vi "UpdateGraphV2.vi"(8 "error in (no error)":errorcluster caption="entrée d'erreur (pas d'erreur)", 10 "GraphIndexArr":i32[](array[numeric]), 11 "Interface en entrée":refnum<class "Interface.lvclass"> caption="DNL_LabVIEW Object in") -> (0 "error out":errorcluster caption="sortie d'erreur", 3 "Interface en sortie":refnum<class "Interface.lvclass"> caption="DNL_LabVIEW Object out")   [LabVIEW 2012, in "Interface.lvclass"]
uses:
  Interface.lvclass
  Interface.lvclass/Interface.ctl
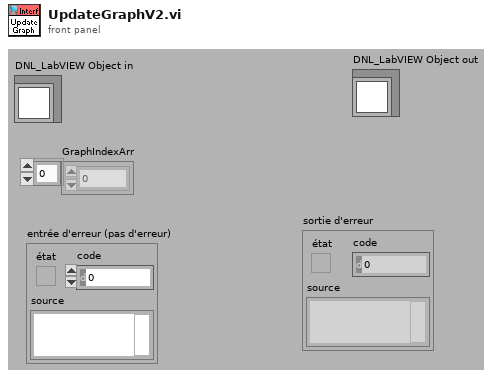
[diagram p1: front panel]
types:
  T1 = typedef "Interface.lvclass/CurveSetup.ctl" = cluster{"CurveName":string, "YParam":string, "XParam":string, "ZParam ":string, "GroupName":string, "LinWdth":u8, "PntCol":u32, "LinCol":u32, "LablFor":u8, "XScale":u32, "YScale":u32, "Interpol":u8, "DisplayName":string, "FillType":i16, "LineStyle":u8, "PntStyle":u8, "BarTyp":u8, "GraphIndex":i32, "Visible":bool, "XScaleName":string, "YScaleName":string, "XYGraph_Ref":refnum<vi>, "Data Only":bool, "DataQ Ref":refnum<queue>, "XParQ Ref":refnum<queue>, "XParamInd":i32, "ScanInd":i32}
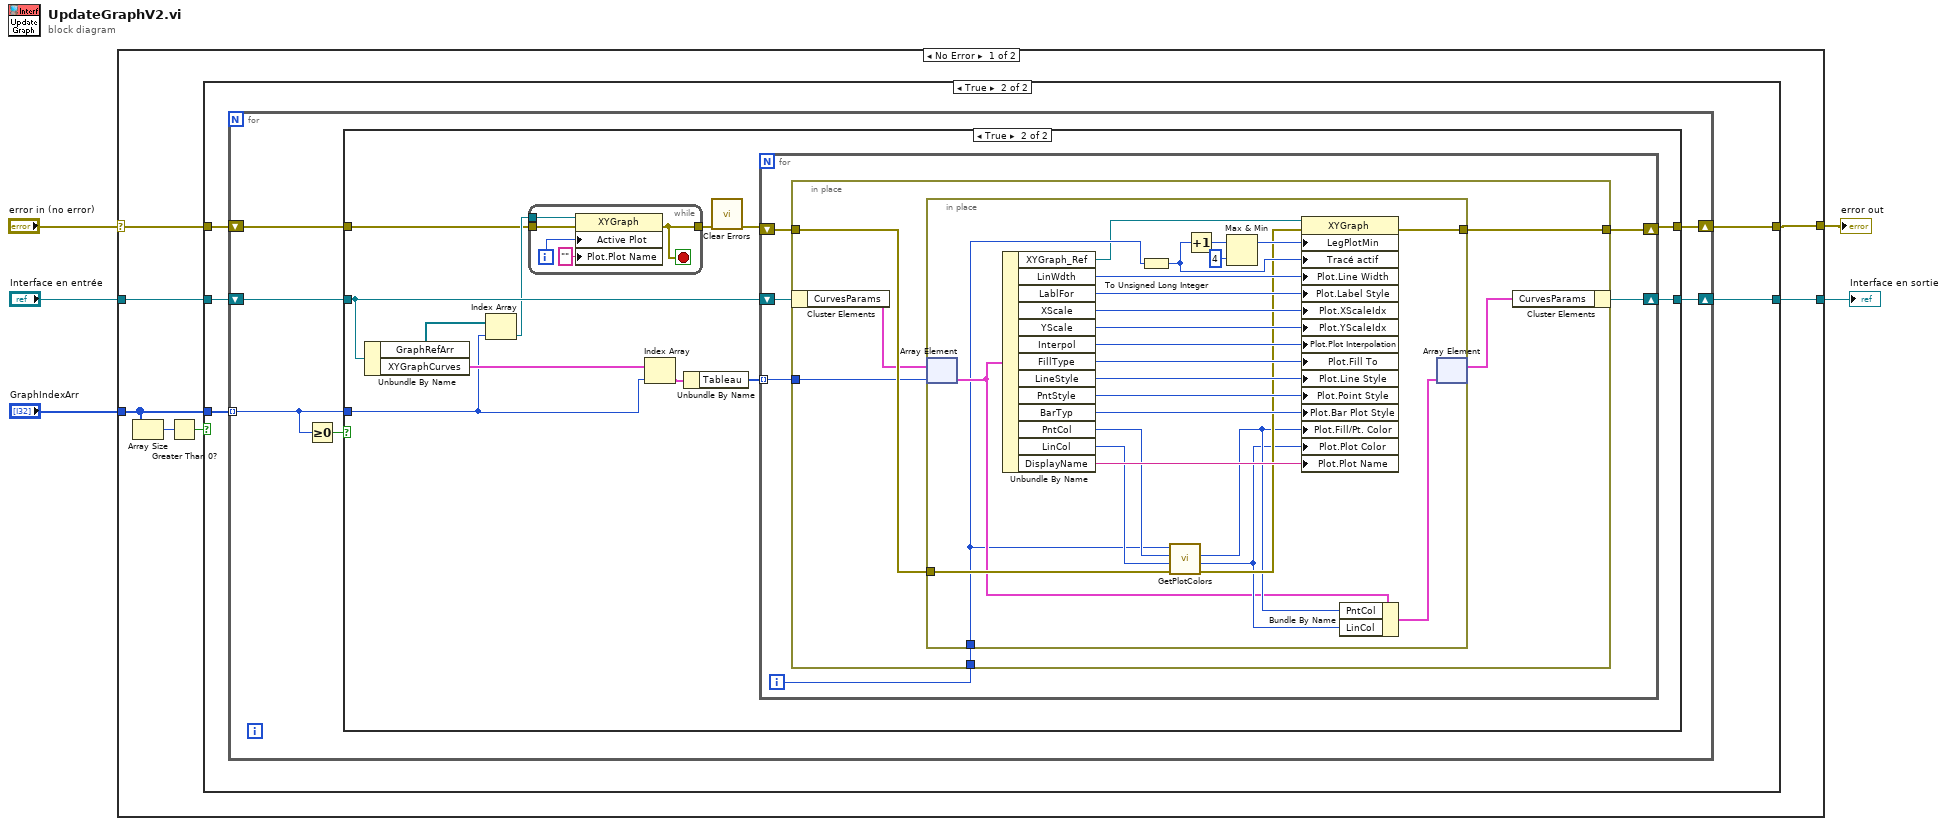
[diagram p0: block diagram]
diagram:
  n1 = case shown="No Error" "error in (no error)" {
    selector: "error in (no error)" -> [w11 w83]
    tunnel: [w12 w83] -> w4
    tunnel: "GraphIndexArr" -> [w9 _]
    tunnel: [w10 w82] -> w1
    tunnel: "Interface en entrée" -> [w6 w82]
    frame No Error {
      n2 = Array Size(array=w9) -> (size(s)=w8:i32)
      n3 = Greater Than 0?(x=w8) -> (x > 0?=w7:bool)
      n4 = case shown="True" w7 {
        tunnel: [w14 w19] -> w12
        tunnel: w9 -> [_ w18]
        tunnel: w11 -> [w14 w17]
        tunnel: [w13 w16] -> w10
        tunnel: w6 -> [w13 w15]
        frame False {
        }
        frame True {
          n5 = for {
            tunnel: w18 -> [w22] mode=indexing
            shift-right: [w25] -> w19
            shift-left: w17 -> [w23]
            shift-right: [w24] -> w16
            shift-left: w15 -> [w20]
            n6 = Greater Or Equal To 0?(x=w22) -> (x >= 0?=w21:bool)
            n7 = case shown="True" w21 {
              tunnel: [w26 w39] -> w25
              tunnel: [w27 w38] -> w24
              tunnel: w22 -> [_ w32]
              tunnel: w20 -> [w27 w35]
              tunnel: w23 -> [w26 w29]
              frame False {
              }
              frame True {
                n8 = Unbundle By Name(w35) -> ("GraphRefArr"=w30:refnum<vi>[], "XYGraphCurves"=w37:cluster{"Tableau":i32[]}[])
                n9 = Index Array(array=w30, index=w32) -> (element=w31:refnum<vi>)
                n10 = while {
                  tunnel: w31 -> [w44]
                  tunnel: w29 -> [w42]
                  tunnel: [w40] -> w33
                  i -> [w41]
                  stop <- w40 stop-if-true
                  n11 = property class="XYGraph"(reference=w44, error in=w42, "Active Plot"=w41, "Plot.Plot Name"="" ("Tracé.Nom du tracé")) -> (error out=w40:errorcluster)  [unwired: 1 out]
                }
                n12 = Index Array(array=w37, index=w32) -> (element=w36:cluster{"Tableau":i32[]})
                n13 = Unbundle By Name(w36) -> ("Tableau"=w34:i32[])
                n14 = call <vilib>:"Clear Errors.vi"("error in (no error)"=w33) -> ("error out"=w28:errorcluster)  [unwired: 6 in]
                n15 = for {
                  shift-right: [w49] -> w38
                  shift-left: w35 -> [w48]
                  tunnel: w34 -> [w47] mode=indexing
                  shift-right: [w50] -> w39
                  shift-left: w28 -> [w45]
                  i -> [w46]
                  n16 = in-place {
                    in-place-border: w45 -> [w56]
                    in-place-border: [w55] -> w50
                    in-place-border: w47 -> [w52]
                    in-place-border: w46 -> [w51]
                    n17 = in-place-cluster #1(w48) -> ("CurvesParams"=w54:T1[])
                    n18 = in-place {
                      in-place-border: [w80] -> w55
                      in-place-border: w56 -> [w64]
                      in-place-border: w51 -> [w58]
                      n19 = in-place-array #2(w54, w52) -> (w60:T1)
                      n20 = Unbundle By Name(w60) -> ("XYGraph_Ref"=w57:refnum<vi>, "LinWdth"=w73:u8, "LablFor"=w74:u8, "XScale"=w72:u32, "YScale"=w71:u32, "Interpol"=w75:u8, "FillType"=w76:i16, "LineStyle"=w77:u8, "PntStyle"=w78:u8, "BarTyp"=w79:u8, "PntCol"=w66:u32, "LinCol"=w65:u32, "DisplayName"=w81:string)
                      n21 = To Unsigned Long Integer(number=w58) -> (unsigned 32bit integer=w67:u32)
                      n22 = call "GetPlotColors.vi"("ErrorIn(No Error)"=w64, "Color2In"=w65, "Color1In"=w66, "ColorIndex"=w58) -> ("sortie d'erreur"=w63:errorcluster, "Color2Out"=w61:u32, "Color1Out"=w62:u32)  [unwired: 4 in, 1 out]
                      n23 = Increment(x=w67) -> (x+1=w70:u32)
                      n24 = Max & Min(x=w70, y=u32 4) -> (max(x,y)=w68:u32)  [unwired: 1 out]
                      n25 = property class="XYGraph"(reference=w57, error in=w63, "LegPlotMin"=w68, "Tracé actif"=w67, "Plot.Line Width"=w73, "Plot.Label Style"=w74, "Plot.XScaleIdx"=w72, "Plot.YScaleIdx"=w71, "Plot.Plot Interpolation"=w75, "Plot.Fill To"=w76, "Plot.Line Style"=w77, "Plot.Point Style"=w78, "Plot.Bar Plot Style"=w79, "Plot.Fill/Pt. Color"=w62, "Plot.Plot Color"=w61, "Plot.Plot Name"=w81) -> (error out=w80:errorcluster)  [unwired: 1 out]
                      n26 = Bundle By Name(cluster=w60, "PntCol"=w62, "LinCol"=w61) -> (w59:T1)
                      n27 = in-place-array #2(w59) -> (w53:T1[])  [unwired: 1 out]
                    }
                    n28 = in-place-cluster #1("CurvesParams"=w53) -> (w49:refnum<class "Interface.lvclass">)
                  }
                }
              }
            }
          }
        }
      }
    }
    frame Error {
    }
  }
  "error out" <- w4
  "Interface en sortie" <- w1
